vi "myRIO v1.1 Open Throughput DI (N Samples).vi"(7 "Allow multiple opens?":bool, 8 "error in (no error)":errorcluster, 10 "Channel Names":string[](array[string]), 11 "Resource name":T3 caption="RIO Device") -> (0 "error out":errorcluster, 2 "DI (N Samples) Channel List":T4, 3 "myRIO Ref Out":T1)   [LabVIEW 2021]
uses:
  <vilib>/myRIO/Common/Instrument Driver Framework/myRIO v1.0/DI Block/typedefs/DI Block Channels List.ctl
  <vilib>/myRIO/Common/Instrument Driver Framework/myRIO v1.0/DI Block/typedefs/DI Block Channels Enum.ctl
  <vilib>/userDefined/High Color/nirio_resource_hc.ctl
  <vilib>/myRIO/Common/Instrument Driver Framework/Utilities/typedefs/myRIO v1.0 Reference.ctl
  <vilib>/myRIO/Common/Instrument Driver Framework/Utilities/typedefs/Generic FPGA Reference.ctl
  <vilib>/Utility/VariantDataType/GetNumericInfo.vi
  <vilib>/Utility/error.llb/Error Cluster From Error Code.vi
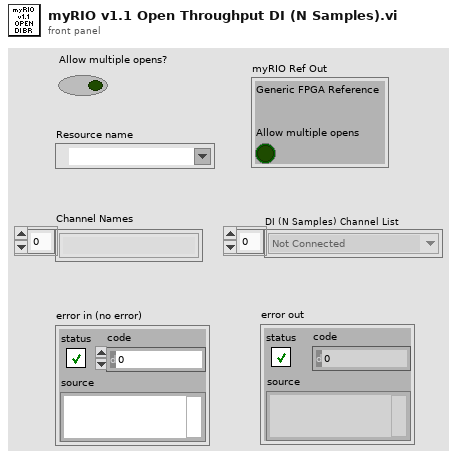
[diagram p1: front panel]
types:
  T1 = typedef "myRIO v1.0 Reference.ctl" = cluster{"Generic FPGA Reference":T2, "Allow multiple opens":bool}
  T2 = typedef "Generic FPGA Reference.ctl" = refnum<k20>
  T3 = typedef "nirio_resource_hc.ctl" = tag
  T4 = typedef "DI Block Channels List.ctl" = T5[]
  T5 = typedef "DI Block Channels Enum.ctl" = enum16{"Not Connected", "A/DI0 (N Samples)", "A/DI1 (N Samples)", "A/DI2 (N Samples)", "A/DI3 (N Samples)", "A/DI4 (N Samples)", "A/DI5 (N Samples)", "A/DI6 (N Samples)", "A/DI7 (N Samples)", "A/DI8 (N Samples)", "A/DI9 (N Samples)", "A/DI10 (N Samples)", "A/DI11 (N Samples)", "A/DI12 (N Samples)", "A/DI13 (N Samples)", "A/DI14 (N Samples)", "A/DI15 (N Samples)", "A/DI16 (N Samples)", "A/DI17 (N Samples)", "A/DI18 (N Samples)", "A/DI19 (N Samples)", "B/DI0 (N Samples)", "B/DI1 (N Samples)", "B/DI2 (N Samples)", "B/DI3 (N Samples)", "B/DI4 (N Samples)", "B/DI5 (N Samples)", "B/DI6 (N Samples)", "B/DI7 (N Samples)", "B/DI8 (N Samples)", "B/DI9 (N Samples)", "B/DI10 (N Samples)", "B/DI11 (N Samples)", "B/DI12 (N Samples)", "B/DI13 (N Samples)", "B/DI14 (N Samples)", "B/DI15 (N Samples)", "B/DI16 (N Samples)", "B/DI17 (N Samples)", "B/DI18 (N Samples)", "B/DI19 (N Samples)"}
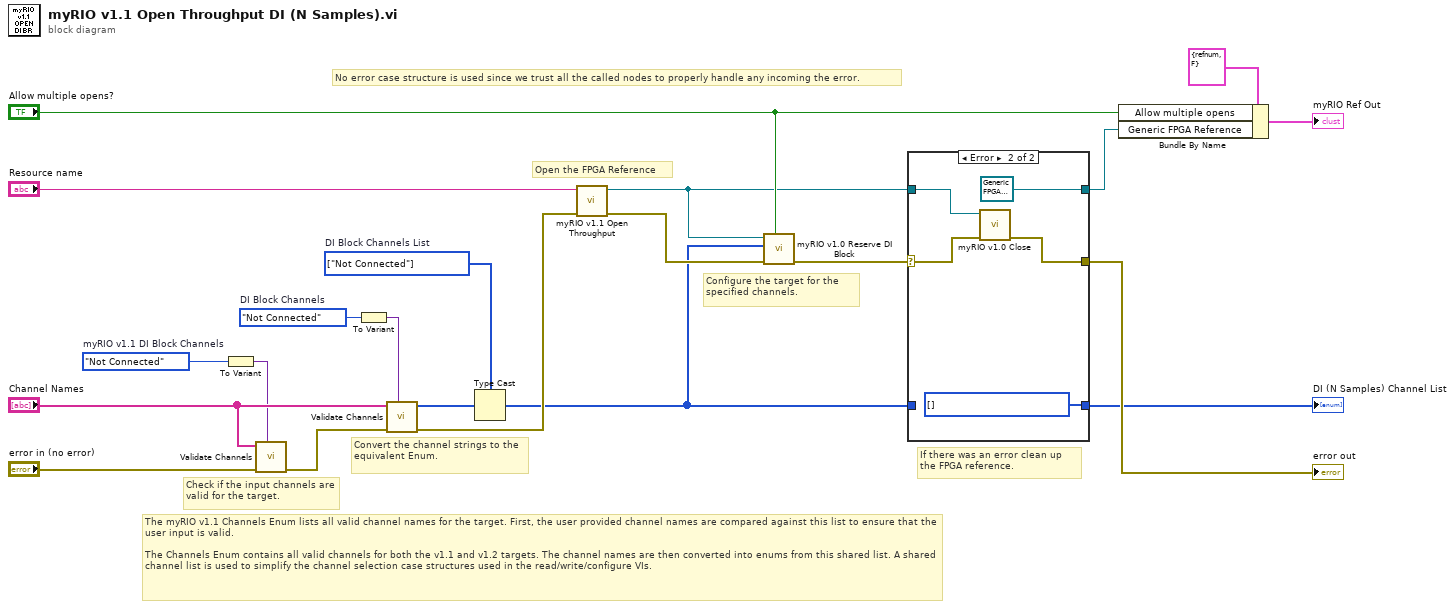
[diagram p0: block diagram]
diagram:
  w4 = DI_Block_Channels_Enum."Not Connected"  # myRIO v1.1 DI Block Channels
  w5 = DI_Block_Channels_Enum."Not Connected"  # DI Block Channels
  w6 = T4 [enum."Not Connected"] items=["Not Connected", "A/DI0 (N Samples)", "A/DI1 (N Samples)", "A/DI2 (N Samples)", "A/DI3 (N Samples)", "A/DI4 (N Samples)", "A/DI5 (N Samples)", "A/DI6 (N Samples)", "A/DI7 (N Samples)", "A/DI8 (N Samples)", "A/DI9 (N Samples)", "A/DI10 (N Samples)", "A/DI11 (N Samples)", "A/DI12 (N Samples)", "A/DI13 (N Samples)", "A/DI14 (N Samples)", "A/DI15 (N Samples)", "A/DI16 (N Samples)", "A/DI17 (N Samples)", "A/DI18 (N Samples)", "A/DI19 (N Samples)", "B/DI0 (N Samples)", "B/DI1 (N Samples)", "B/DI2 (N Samples)", "B/DI3 (N Samples)", "B/DI4 (N Samples)", "B/DI5 (N Samples)", "B/DI6 (N Samples)", "B/DI7 (N Samples)", "B/DI8 (N Samples)", "B/DI9 (N Samples)", "B/DI10 (N Samples)", "B/DI11 (N Samples)", "B/DI12 (N Samples)", "B/DI13 (N Samples)", "B/DI14 (N Samples)", "B/DI15 (N Samples)", "B/DI16 (N Samples)", "B/DI17 (N Samples)", "B/DI18 (N Samples)", "B/DI19 (N Samples)"]  # DI Block Channels List
  # "The myRIO v1.1 Channels Enum lists all valid channel names for the target. First, the user provided channel names are compared against this list to ensure that the user input is valid.\n\nThe Channels Enum contains all valid channels for both the v1.1 and v1.2 targets. The channel names are then converted into enums from this shared list. A shared channel list is used to simplify the channel selection case structures used in the read/write/configure VIs."
  # "If there was an error clean up the FPGA reference."
  # "Configure the target for the specified channels."
  # "Open the FPGA Reference"
  # "No error case structure is used since we trust all the called nodes to properly handle any incoming the error."
  # "Convert the channel strings to the equivalent Enum."
  # "Check if the input channels are valid for the target."
  n1 = To Variant(anything=w4) -> (Variant=w7:variant)
  n2 = call <vilib>:"Validate Channels.vi"("Channels Enum Variant"=w7, "error in (no error)"="error in (no error)", "Channel Names"="Channel Names") -> ("error out"=w20:errorcluster)  [unwired: 7 in, 1 out]
  n3 = To Variant(anything=w5) -> (Variant=w8:variant)
  n4 = call <vilib>:"Validate Channels.vi"("Channels Enum Variant"=w8, "error in (no error)"=w20, "Channel Names"="Channel Names") -> ("error out"=w16:errorcluster, "Index Array"=w15:u16[])  [unwired: 7 in]
  n5 = Type Cast(type=w6, x=w15) -> (*(type *) &x=w12:T4)
  n6 = call <vilib>:"myRIO v1.1 Open Throughput.vi"("error in (no error)"=w16, "Resource name"="Resource name") -> ("error out"=w14:errorcluster, "myRIO FPGA Ref Out"=w1:T2)  [unwired: 8 in]
  n7 = call <vilib>:"myRIO v1.0 Reserve DI Block.vi"("Allow multiple opens?"="Allow multiple opens?", "error in (no error)"=w14, "DI (N Samples) Channel List"=w12, "Generic FPGA Reference"=w1) -> ("error out"=w13:errorcluster)  [unwired: 7 in]
  n8 = case shown="Error" w13 {
    selector: w13 -> [w23 w29]
    tunnel: w1 -> [w24 w27]
    tunnel: [w24 T2 refnum ("myRIO FPGA Ref Out")] -> w9
    tunnel: [w23 w28] -> w18
    tunnel: w12 -> [w22 _]
    tunnel: [w22 w25] -> w11
    frame No Error {
    }
    frame Error {
      w25 = T4 [] items=["Not Connected", "A/DI0 (N Samples)", "A/DI1 (N Samples)", "A/DI2 (N Samples)", "A/DI3 (N Samples)", "A/DI4 (N Samples)", "A/DI5 (N Samples)", "A/DI6 (N Samples)", "A/DI7 (N Samples)", "A/DI8 (N Samples)", "A/DI9 (N Samples)", "A/DI10 (N Samples)", "A/DI11 (N Samples)", "A/DI12 (N Samples)", "A/DI13 (N Samples)", "A/DI14 (N Samples)", "A/DI15 (N Samples)", "A/DI16 (N Samples)", "A/DI17 (N Samples)", "A/DI18 (N Samples)", "A/DI19 (N Samples)", "B/DI0 (N Samples)", "B/DI1 (N Samples)", "B/DI2 (N Samples)", "B/DI3 (N Samples)", "B/DI4 (N Samples)", "B/DI5 (N Samples)", "B/DI6 (N Samples)", "B/DI7 (N Samples)", "B/DI8 (N Samples)", "B/DI9 (N Samples)", "B/DI10 (N Samples)", "B/DI11 (N Samples)", "B/DI12 (N Samples)", "B/DI13 (N Samples)", "B/DI14 (N Samples)", "B/DI15 (N Samples)", "B/DI16 (N Samples)", "B/DI17 (N Samples)", "B/DI18 (N Samples)", "B/DI19 (N Samples)"] ("DIO Channels List")
      n9 = call <vilib>:"myRIO v1.0 Close.vi"("error in (no error)"=w29, "myRIO FPGA Ref In"=w27) -> ("error out"=w28:errorcluster)  [unwired: 9 in]
    }
  }
  "DI (N Samples) Channel List" <- w11
  "error out" <- w18
  n10 = Bundle By Name(cluster=T1 {"Generic FPGA Reference"=refnum, "Allow multiple opens"=FALSE} ("myRIO Ref Out"), "Allow multiple opens"="Allow multiple opens?", "Generic FPGA Reference"=w9) -> (→"myRIO Ref Out":T1)
